vi "MB Ethernet Is Address Valid.vi"(8 "error in (no error)":errorcluster, 10 "Valid IP Addresses":string[](array[string]), 11 "IP Address":string) -> (0 "error out":errorcluster, 3 "IP Valid":bool)   [LabVIEW 2019, in "NI_modbus_upd.lvlib"]
uses:
  NI_modbus_upd.lvlib
panel:
  # "VI Name: MB Ethernet Is Address Valid.vi\nPurpose: Verifies if the IP Address can be masked by one of the\naddresses provided in the Valid IP Addresses array."
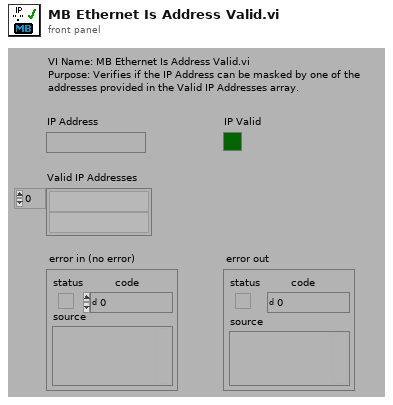
[diagram p1: front panel]
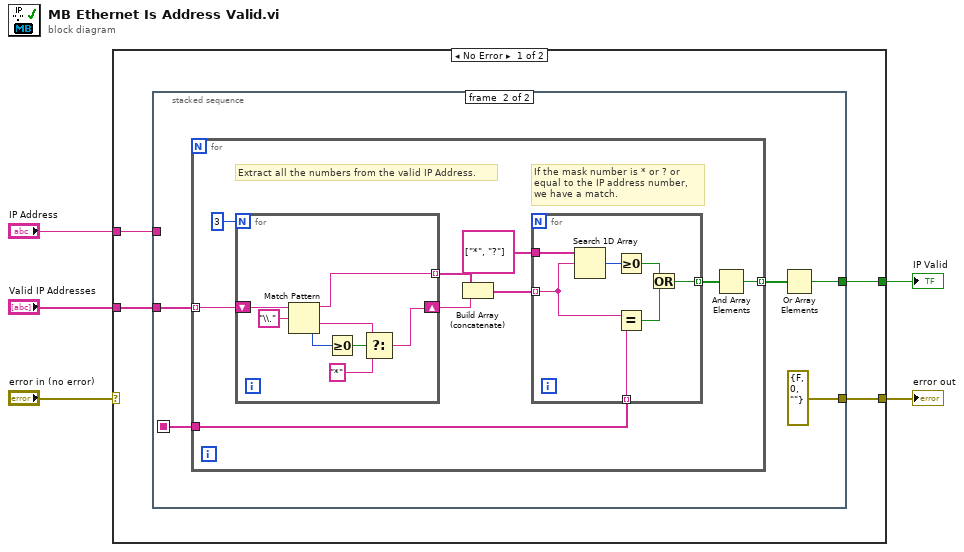
[diagram p0: block diagram]
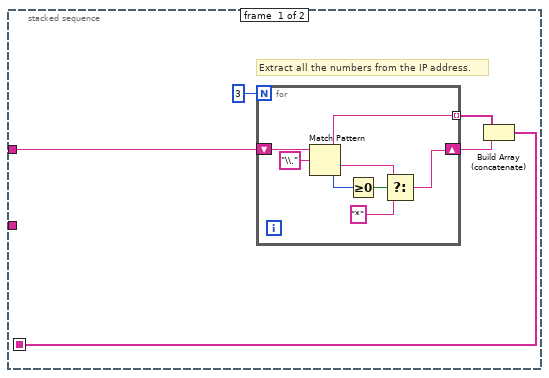
[diagram p2: hidden frame]
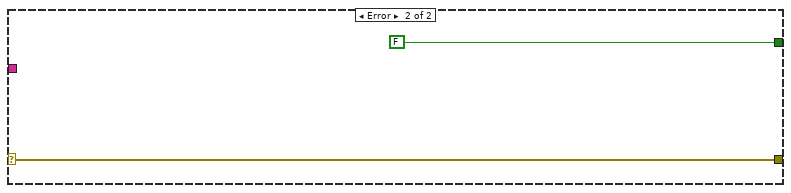
[diagram p3: hidden frame]
diagram:
  n1 = case shown="No Error" "error in (no error)" {
    selector: "error in (no error)" -> [_ w52]
    tunnel: "Valid IP Addresses" -> [w9 _]
    tunnel: "IP Address" -> [w6 _]
    tunnel: [w8 FALSE] -> w3
    tunnel: [w7 w52] -> w1
    frame No Error {
      n2 = stacked-sequence {
        seq-local: [w11 _] -> [_ w23]
        tunnel: w9 -> [_ w27]
        tunnel: [_ w26] -> w8
        tunnel: [_ errorcluster {"status"=FALSE, "code"=0, "source"=""} ("error IO")] -> w7
        tunnel: w6 -> [w10 _]
        frame #0 {
          # "Extract all the numbers from the IP address."
          n3 = for {
            N: 3 -> [_]
            shift-right: [w16] -> w13
            shift-left: w10 -> [w22]
            tunnel: [w15] -> w12 mode=indexing
            n4 = Match Pattern(string=w22, regular expression="\\.") -> (before substring=w15:string, after substring=w18:string, offset past match=w20:i32)  [unwired: 1 in, 1 out]
            n5 = Greater Or Equal To 0?(x=w20) -> (x >= 0?=w19:bool)
            n6 = Select(t=w18, s=w19, f="*") -> (s? t:f=w16:string)
          }
          n7 = Build Array (concatenate)(w12, w13) -> (w11:string[])
        }
        frame #1 {
          n8 = for {
            tunnel: w27 -> [w36] mode=indexing
            tunnel: [w29] -> w25 mode=indexing
            tunnel: w23 -> [w28]
            # "If the mask number is * or ? or equal to the IP address number, we have a match."
            # "Extract all the numbers from the valid IP Address."
            n9 = for {
              N: 3 -> [_]
              shift-right: [w45] -> w34
              shift-left: w36 -> [w51]
              tunnel: [w44] -> w33 mode=indexing
              n10 = Match Pattern(string=w51, regular expression="\\.") -> (before substring=w44:string, after substring=w47:string, offset past match=w49:i32)  [unwired: 1 in, 1 out]
              n11 = Greater Or Equal To 0?(x=w49) -> (x >= 0?=w48:bool)
              n12 = Select(t=w47, s=w48, f="*") -> (s? t:f=w45:string)
            }
            n13 = Build Array (concatenate)(w33, w34) -> (w30:string[])
            n14 = for {
              tunnel: [w39] -> w31 mode=indexing
              tunnel: string[] ["*", "?"] -> [w42]
              tunnel: w30 -> [w38] mode=indexing
              tunnel: w28 -> [w37] mode=indexing
              n15 = Search 1D Array(1D array=w42, element=w38) -> (index of element=w43:i32)  [unwired: 1 in]
              n16 = Greater Or Equal To 0?(x=w43) -> (x >= 0?=w41:bool)
              n17 = Equal?(x=w38, y=w37) -> (x = y?=w40:bool)
              n18 = Or(x=w41, y=w40) -> (x .or. y?=w39:bool)
            }
            n19 = And Array Elements(Boolean array=w31) -> (logical AND=w29:bool)
          }
          n20 = Or Array Elements(Boolean array=w25) -> (logical OR=w26:bool)
        }
      }
    }
    frame Error {
    }
  }
  "IP Valid" <- w3
  "error out" <- w1
